vi "myRIO v1.0 DI Block Read.vi"(7 "DI FIFO Sample Rate (Hz)":dbl=1000.0 min=1000.0 max=8000000.0, 8 "error in (no error)":errorcluster, 9 "Number of Samples":u32=1000, 10 "DI (N Samples) Channel List":T3, 11 "myRIO Ref In":T1) -> (0 "error out":errorcluster, 2 "bool Value List":bool[][](array[boolean]), 3 "myRIO Ref Out":T1)   [LabVIEW 2021]
uses:
  <vilib>/myRIO/Common/Instrument Driver Framework/myRIO v1.0/DI Block/typedefs/DI Block Channels List.ctl
  <vilib>/myRIO/Common/Instrument Driver Framework/myRIO v1.0/DI Block/typedefs/DI Block Channels Enum.ctl
  <vilib>/myRIO/Common/Instrument Driver Framework/Utilities/typedefs/myRIO v1.0 Reference.ctl
  <vilib>/myRIO/Common/Instrument Driver Framework/Utilities/typedefs/Generic FPGA Reference.ctl
  <vilib>/myRIO/Common/Instrument Driver Framework/myRIO v1.0/DI Block/typedefs/DI Block FPGA Reference.ctl
  <vilib>/myRIO/Common/Instrument Driver Framework/myRIO v1.0/Resource Manager/vis/myRIO v1.0 Block Write Configuration.vi
  <vilib>/rvi/errors/niLvFpgaAdjustHostInterfaceError.vi
  <vilib>/rvi/interface/nirviMethod/nirviMethod.xnode
  <vilib>/rvi/interface/nirviReadWriteControl/nirviReadWriteControl.xnode
  <vilib>/rvi/errors/niLvFpgaMergeErrorWithErrorCode.vi
  <vilib>/rvi/interface/Simulation/niFpgaSimulationCallBeginRW.vi
  NiFpgaLv.dll
  <vilib>/FPGAPlugInAG/Dynamic/niLvFpga_StartFifo_Dynamic.vi
  <vilib>/FPGAPlugInAG/Dynamic/niLvFpga_StopFifo_Dynamic.vi
  <vilib>/FPGAPlugInAG/Dynamic/niLvFpga_ReadFifo_Dynamic.vi
panel:
  # "This VI reads boolean values from a list of user specified channels on\nthe myRIO v1.0 hardware. The values are read on the FPGA as a bit and \nconverted to a boolean. Please see Block Diagram for details."
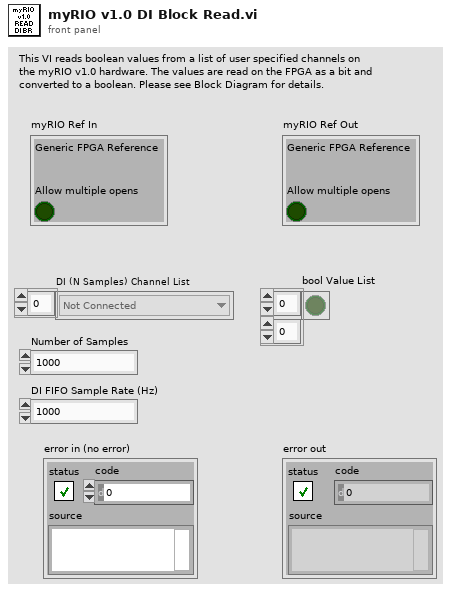
[diagram p1: front panel]
types:
  T1 = typedef "myRIO v1.0 Reference.ctl" = cluster{"Generic FPGA Reference":T2, "Allow multiple opens":bool}
  T2 = typedef "Generic FPGA Reference.ctl" = refnum<k20>
  T3 = typedef "DI Block Channels List.ctl" = T4[]
  T4 = typedef "DI Block Channels Enum.ctl" = enum16{"Not Connected", "A/DI0 (N Samples)", "A/DI1 (N Samples)", "A/DI2 (N Samples)", "A/DI3 (N Samples)", "A/DI4 (N Samples)", "A/DI5 (N Samples)", "A/DI6 (N Samples)", "A/DI7 (N Samples)", "A/DI8 (N Samples)", "A/DI9 (N Samples)", "A/DI10 (N Samples)", "A/DI11 (N Samples)", "A/DI12 (N Samples)", "A/DI13 (N Samples)", "A/DI14 (N Samples)", "A/DI15 (N Samples)", "A/DI16 (N Samples)", "A/DI17 (N Samples)", "A/DI18 (N Samples)", "A/DI19 (N Samples)", "B/DI0 (N Samples)", "B/DI1 (N Samples)", "B/DI2 (N Samples)", "B/DI3 (N Samples)", "B/DI4 (N Samples)", "B/DI5 (N Samples)", "B/DI6 (N Samples)", "B/DI7 (N Samples)", "B/DI8 (N Samples)", "B/DI9 (N Samples)", "B/DI10 (N Samples)", "B/DI11 (N Samples)", "B/DI12 (N Samples)", "B/DI13 (N Samples)", "B/DI14 (N Samples)", "B/DI15 (N Samples)", "B/DI16 (N Samples)", "B/DI17 (N Samples)", "B/DI18 (N Samples)", "B/DI19 (N Samples)"}
  T5 = typedef "DI Block FPGA Reference.ctl" = refnum<k20>
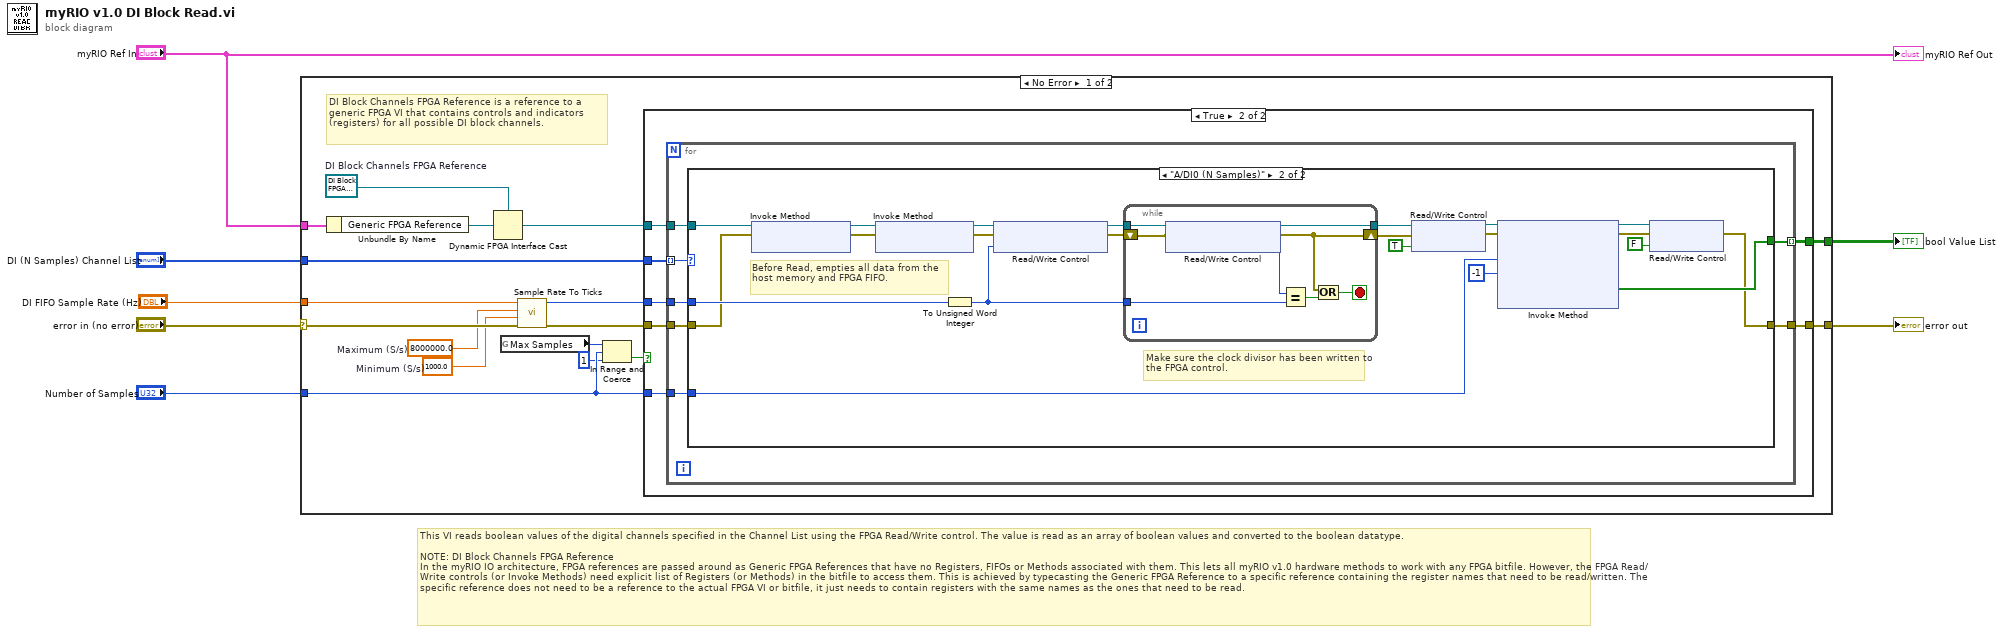
[diagram p0: block diagram]
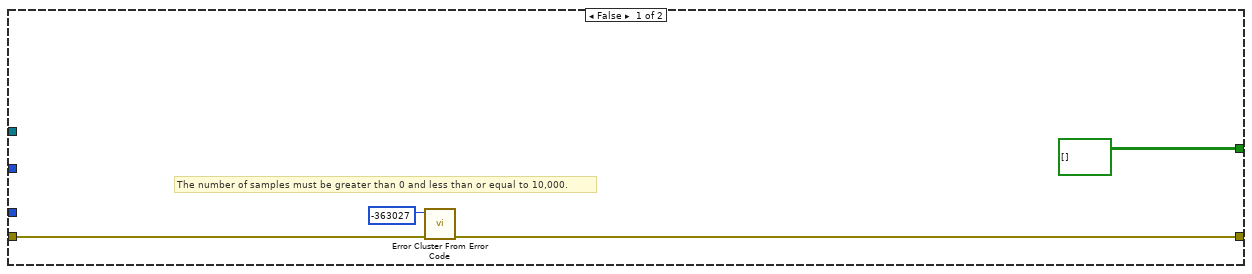
[diagram p2: hidden frame]
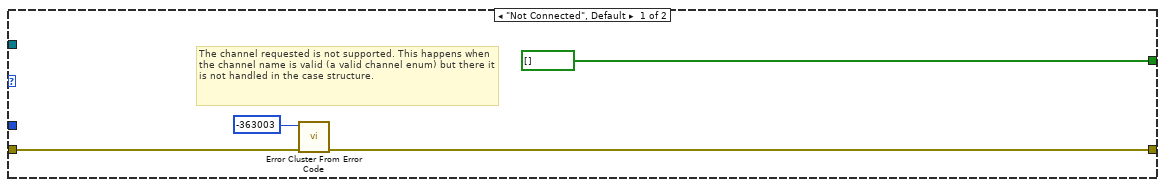
[diagram p3: hidden frame]
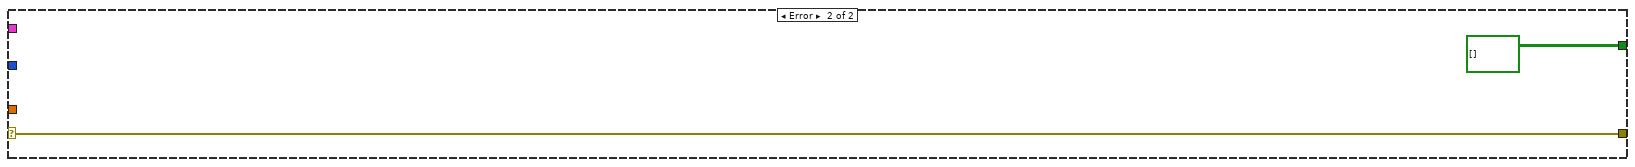
[diagram p4: hidden frame]
diagram:
  # "This VI reads boolean values of the digital channels specified in the Channel List using the FPGA Read/Write control. The value is read as an array of boolean values and converted to the boolean datatype. \n\nNOTE: DI Block Channels FPGA Reference\nIn the myRIO IO architecture, FPGA references are passed around as Generic FPGA References that have no Registers, FIFOs or Methods associated with them. This lets all myRIO v1.0 hardware methods to work with any FPGA bitfile. However, the FPGA Read/Write controls (or Invoke Methods) need explicit list of Registers (or Methods) in the bitfile to access them. This is achieved by typecasting the Generic FPGA Reference to a specific reference containing the register names that need to be read/written. The specific reference does not need to be a reference to the actual FPGA VI or bitfile, it just needs to contain registers with the same names as the ones that need to be read."
  n1 = case shown="No Error" "error in (no error)" {
    selector: "error in (no error)" -> [w14 w78]
    tunnel: "myRIO Ref In" -> [w23 _]
    tunnel: [w18 w78] -> w7
    tunnel: [w20 bool[][] []] -> w5
    tunnel: "DI (N Samples) Channel List" -> [w21 _]
    tunnel: "Number of Samples" -> [w10 _]
    tunnel: "DI FIFO Sample Rate (Hz)" -> [w15 _]
    frame No Error {
      w12 = 1000.0  # Minimum (S/s)
      w13 = 8000000.0  # Maximum (S/s)
      w24 = T5 refnum  # DI Block Channels FPGA Reference
      # "DI Block Channels FPGA Reference is a reference to a generic FPGA VI that contains controls and indicators (registers) for all possible DI block channels."
      n2 = Unbundle By Name(w23) -> ("Generic FPGA Reference"=w22:T2)
      n3 = Dynamic FPGA Interface Cast(Session In=w24, Type=w22) -> (Session Out=w19:T5)
      n4 = global read "myRIO v1.0 Block Write Configuration.vi" "Max Samples"() -> (w11:u32)
      n5 = call <vilib>:"Sample Rate To Ticks.vi"("error in (no error)"=w14, "Minimum (S/s)"=w12, "Maximum (S/s)"=w13, "Sample Rate (S/s)"=w15) -> ("error out"=w16:errorcluster, "Count (tick/s)"=w17:u32)  [unwired: 5 in, 1 out]
      n6 = In Range and Coerce(upper limit=w11, x=w10, lower limit=u32 1) -> (In Range?=w8:bool)  [unwired: 1 out]
      n7 = case shown="True" w8 {
        tunnel: w16 -> [w27 w35]
        tunnel: w21 -> [_ w34]
        tunnel: [bool[][] [] ("Data") w33] -> w20
        tunnel: w19 -> [_ w32]
        tunnel: w17 -> [_ w31]
        tunnel: [w26 w30] -> w18
        tunnel: w10 -> [_ w29]
        frame False {
          # "The number of samples must be greater than 0 and less than or equal to 10,000."
          n8 = call <vilib>:"Error Cluster From Error Code.vi"("error in (no error)"=w27, "error code (0)"=-363027) -> ("error out"=w26:errorcluster)  [unwired: 7 in]
        }
        frame True {
          n9 = for {
            tunnel: w34 -> [w42] mode=indexing
            tunnel: w35 -> [w39]
            tunnel: [w41] -> w33 mode=indexing
            tunnel: w32 -> [w40]
            tunnel: w29 -> [w38]
            tunnel: w31 -> [w37]
            tunnel: [w36] -> w30
            n10 = case shown="\"A/DI0 (N Samples)\"" w42 {
              tunnel: [bool[] [] w48] -> w41
              tunnel: w40 -> [_ w67]
              tunnel: w39 -> [w45 w59]
              tunnel: w38 -> [_ w53]
              tunnel: w37 -> [_ w68]
              tunnel: [w44 w47] -> w36
              frame "Not Connected", Default {
                # "The channel requested is not supported. This happens when the channel name is valid (a valid channel enum) but there it is not handled in the case structure."
                n11 = call <vilib>:"Error Cluster From Error Code.vi"("error in (no error)"=w45, "error code (0)"=-363003) -> ("error out"=w44:errorcluster)  [unwired: 7 in]
              }
              frame "A/DI0 (N Samples)" {
                # "Make sure the clock divisor has been written to the FPGA control."
                # "Before Read, empties all data from the host memory and FPGA FIFO."
                n12 = xnode "Invoke Method"("FPGA VI Reference In"=w67, "error in"=w59) -> ("FPGA VI Reference Out"=w66:T5, "error out"=w65:errorcluster)
                n13 = xnode "Invoke Method"("FPGA VI Reference In"=w66, "error in"=w65) -> ("FPGA VI Reference Out"=w64:T5, "error out"=w63:errorcluster)
                n14 = To Unsigned Word Integer(number=w68) -> (unsigned 16bit integer=w62:u16)
                n15 = xnode "Read/Write Control"("FPGA VI Reference In"=w64, "error in"=w63, "DI.A_0.ClockDivisor"=w62) -> ("FPGA VI Reference Out"=w61:T5, "error out"=w60:errorcluster)
                n16 = while {
                  tunnel: w61 -> [w73]
                  tunnel: [w71] -> w58
                  shift-right: [w70] -> w57
                  shift-left: w60 -> [w69]
                  tunnel: w62 -> [w76]
                  stop <- w74 stop-if-true
                  n17 = xnode "Read/Write Control"("FPGA VI Reference In"=w73, "error in"=w69) -> ("FPGA VI Reference Out"=w71:T5, "error out"=w70:errorcluster, "DI.A_0.ClockDivisor"=w72:u16)
                  n18 = Equal?(x=w72, y=w76) -> (x = y?=w75:bool)
                  n19 = Or(x=w70, y=w75) -> (x .or. y?=w74:bool)
                }
                n20 = xnode "Read/Write Control"("FPGA VI Reference In"=w58, "error in"=w57, "DI.A_0.ENA"=TRUE ("Flag_DI")) -> ("FPGA VI Reference Out"=w55:T5, "error out"=w54:errorcluster)
                n21 = xnode "Invoke Method"("FPGA VI Reference In"=w55, "error in"=w54, "Number of Elements"=w53, "Timeout (ms)"=-1) -> ("FPGA VI Reference Out"=w51:T5, "error out"=w50:errorcluster, "Data"=w48:bool[])  [unwired: 1 out]
                n22 = xnode "Read/Write Control"("FPGA VI Reference In"=w51, "error in"=w50, "DI.A_0.ENA"=FALSE ("Flag")) -> ("error out"=w47:errorcluster)  [unwired: 1 out]
              }
            }
          }
        }
      }
    }
    frame Error {
    }
  }
  "error out" <- w7
  "bool Value List" <- w5
  "myRIO Ref Out" <- "myRIO Ref In"
